vi "Message.vi"(8 "error in (no error)":errorcluster, 9 "Payload":string, 10 "Command":string, 11 "GRPCClient in":refnum<class "MicronGRPCClient.lvclass">) -> (0 "error out":errorcluster, 2 "Response":string, 3 "GRPCClient out":refnum<class "MicronGRPCClient.lvclass">)   [LabVIEW 2019, in "MicronGRPCClient.lvclass"]
uses:
  MicronGRPCClient.lvclass
  Generated/MicronGRPCGeneratedClient/RPC Messages/micronGrpc_MessageRequest.ctl
  MicronGRPCClient.lvclass/MicronGRPCClient.ctl
  06dfe680-f955-41ec-ac1b-feaf7bba287b.vi
  Generated/MicronGRPCGeneratedClient/MicronGRPCGeneratedClient.lvlib
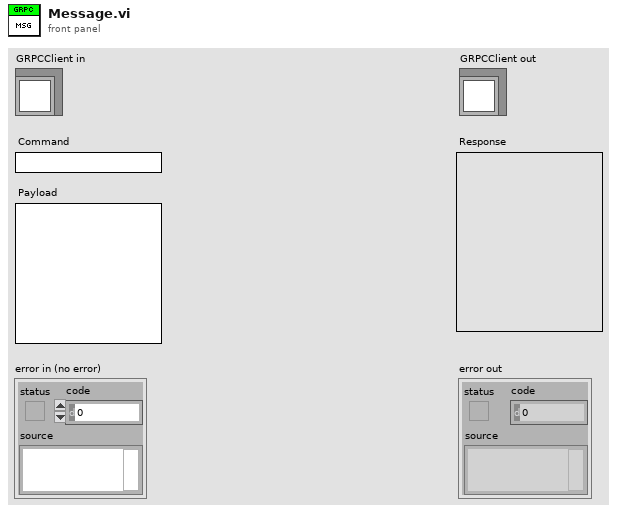
[diagram p1: front panel]
types:
  T1 = typedef "MicronGRPCGeneratedClient.lvlib/micronGrpc_MessageRequest.ctl" = cluster{"command":string, "payload":string}
  T2 = typedef "grpc-lvsupport-release.lvlib/grpcId.ctl" = u64
  T3 = typedef "MicronGRPCGeneratedClient.lvlib/micronGrpc_MessageReply.ctl" = cluster{"payload":string, "status":T4}
  T4 = typedef "MicronGRPCGeneratedClient.lvlib/micronGrpc_MessageReply_Status.ctl" = cluster{"code":i32, "is_error":bool, "desc":string}
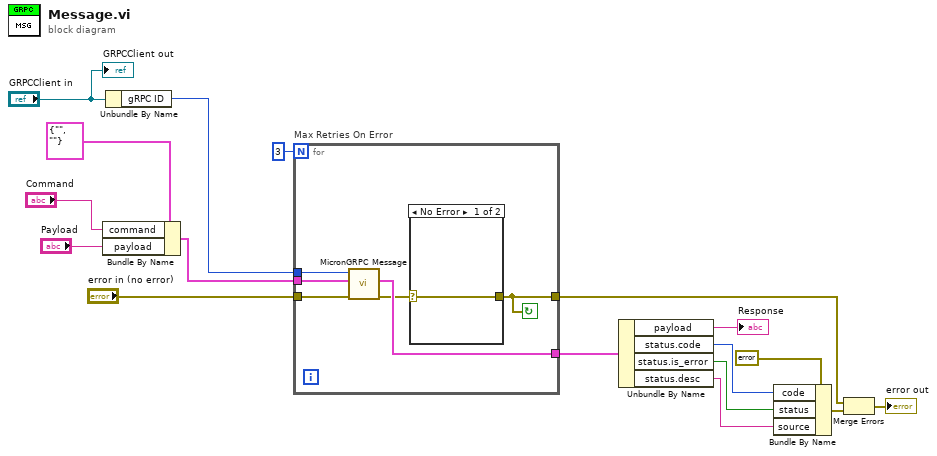
[diagram p0: block diagram]
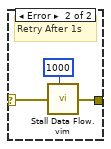
[diagram p2: hidden frame]
diagram:
  n1 = Bundle By Name(cluster=T1 {"command"="", "payload"=""} ("Request Data"), "command"="Command", "payload"="Payload") -> (w9:T1)
  n2 = Unbundle By Name("GRPCClient in") -> ("gRPC ID"=w17:T2)
  n3 = for "Max Retries On Error" {
    N: 3 -> [_]
    tunnel: w17 -> [w23]
    tunnel: [w21] -> w14
    tunnel: w9 -> [w20]
    tunnel: "error in (no error)" -> [w22]
    tunnel: [w18] -> w4
    stop <- w18 continue-if-true
    n4 = call "MicronGRPC Message.vi"("error in"=w22, "Request Data"=w20, "gRPC ID"=w23) -> ("error out"=w19:errorcluster, "Response Data"=w21:T3)  [unwired: 6 in, 1 out]
    n5 = case shown="No Error" w19 {
      selector: w19 -> [w24 w27]
      tunnel: [w24 w26] -> w18
      frame No Error {
      }
      frame Error {
        # "Retry After 1s"
        n6 = call "Stall Data Flow.vim"("value in"=w27, "milliseconds to wait"=u32 1000) -> ("value out"=w26:errorcluster)  [unwired: 1 out]
      }
    }
  }
  n7 = Unbundle By Name(w14) -> ("payload"=→"Response":string, "status.code"=w7:i32, "status.is_error"=w6:bool, "status.desc"=w5:string)
  n8 = Bundle By Name(cluster=errorcluster {"status"=FALSE, "code"=0, "source"=""} ("error out"), "code"=w7, "status"=w6, "source"=w5) -> (w3:errorcluster)
  n9 = Merge Errors(w4, w3) -> (→"error out":errorcluster)
  "GRPCClient out" <- "GRPCClient in"
